vi "Control Drive Motors.vi"(10 "Disable Motors":bool=TRUE, 11 "Cluster":cluster{"RR":dbl, "FR":dbl, "RL":dbl, "FL":dbl}) -> ()   [LabVIEW 2018]
uses:
  <vilib>/Rock Robotics/WPI/Utilities/WPI_GetSetVariantRefNum.vi
  <vilib>/Rock Robotics/Network Tables/NT Write Number.vi
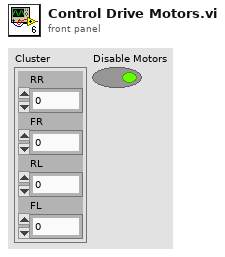
[diagram p1: front panel]
types:
  T1 = typedef "WPI_RobotDriveDevRef.ctl" = cluster{"DevStatus":errorcluster, "Motors[]":T2[], "Square Inputs":bool, "Max Output":dbl}
  T2 = typedef "WPI_MotorControlDeviceRef.ctl" = cluster{"DeviceStatus":errorcluster, "Type":T3, "PWM":cluster{"PWM Channel":T4, "DeadBand":T5}, "CAN":cluster{"Device Number":u8, "SetOutput VI Ref":variant, "GetOutput VI Ref":variant, "Enable VI Ref":variant, "Disable VI Ref":variant, "Data":variant}, "Invert":bool, "DIO PWM":cluster{"PWM \"Enable\" Channel":T4, "DIOChannel":T6, "PWM Rate":dbl}}
  T3 = typedef "WPI_MotorControlType.ctl" = enum16{"PWM", "CAN", "DIO PWM"}
  T4 = typedef "FPGA_DIOPWMChannel.ctl" = enum8{"PWM 0", "PWM 1", "PWM 2", "PWM 3", "PWM 4", "PWM 5", "PWM 6", "PWM 7", "PWM 8", "PWM 9", "PWM MXP 0", "PWM MXP 1", "PWM MXP 2", "PWM MXP 3", "PWM MXP 4", "PWM MXP 5", "PWM MXP 6", "PWM MXP 7", "PWM MXP 8", "PWM MXP 9", "Invalid"}
  T5 = typedef "WPI_PWMDeadband.ctl" = cluster{"Name":string, "maxPositivePwm":i32, "minPositivePwm":i32, "centerPwm":i32, "maxNegativePwm":i32, "minNegativePwm":i32, "angularRange":u16}
  T6 = typedef "FPGA_DIOChannel.ctl" = enum8{"DIO 0", "DIO 1", "DIO 2", "DIO 3", "DIO 4", "DIO 5", "DIO 6", "DIO 7", "DIO 8", "DIO 9", "DIO MXP 0", "DIO MXP 1", "DIO MXP 2", "DIO MXP 3", "DIO MXP 4", "DIO MXP 5", "DIO MXP 6", "DIO MXP 7", "DIO MXP 8", "DIO MXP 9", "DIO MXP 10", "DIO MXP 11", "DIO MXP 12", "DIO MXP 13", "DIO MXP 14", "DIO MXP 15", "SPI Port CS1", "SPI Port CS2", "SPI Port CS3", "SPI Port MISO", "SPI Port MOSI", "Invalid"}
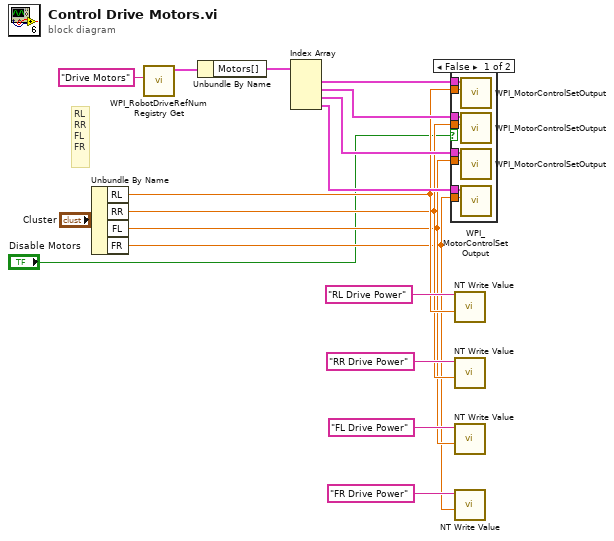
[diagram p0: block diagram]
diagram:
  # "RL\nRR\nFL\nFR"
  n1 = Unbundle By Name("Cluster") -> ("RL"=w5:dbl, "RR"=w4:dbl, "FL"=w3:dbl, "FR"=w2:dbl)
  n2 = call <vilib>:"WPI_RobotDriveRefNum Registry Get.vi"("refnum name"="Drive Motors") -> ("RobotDriveDevRef"=w17:T1)  [unwired: 9 in, 1 out]
  n3 = Unbundle By Name(w17) -> ("Motors[]"=w15:T2[])
  n4 = Index Array(array=w15) -> (element #1=w14:T2, element #2=w13:T2, element #3=w12:T2, element #4=w11:T2)  [unwired: 4 in]
  n5 = case shown="False" "Disable Motors" {
    tunnel: w14 -> [w25 _]
    tunnel: w13 -> [w24 _]
    tunnel: w12 -> [w23 _]
    tunnel: w11 -> [w22 _]
    tunnel: w5 -> [w21 _]
    tunnel: w4 -> [w20 _]
    tunnel: w3 -> [w19 _]
    tunnel: w2 -> [w18 _]
    frame False {
      n6 = call <vilib>:"WPI_MotorControlSetOutput.vi"("Output"=w21, "MotorControlDevRef"=w25) -> ()  [unwired: 7 in, 3 out]
      n7 = call <vilib>:"WPI_MotorControlSetOutput.vi"("Output"=w20, "MotorControlDevRef"=w24) -> ()  [unwired: 7 in, 3 out]
      n8 = call <vilib>:"WPI_MotorControlSetOutput.vi"("Output"=w19, "MotorControlDevRef"=w23) -> ()  [unwired: 7 in, 3 out]
      n9 = call <vilib>:"WPI_MotorControlSetOutput.vi"("Output"=w18, "MotorControlDevRef"=w22) -> ()  [unwired: 7 in, 3 out]
    }
    frame True {
    }
  }
  n10 = call-poly <vilib>:"NT Write Value.vi"("Numeric"=w5, "Name"="RL Drive Power") -> ()  [unwired: 9 in, 1 out]
  n11 = call-poly <vilib>:"NT Write Value.vi"("Numeric"=w4, "Name"="RR Drive Power") -> ()  [unwired: 9 in, 1 out]
  n12 = call-poly <vilib>:"NT Write Value.vi"("Numeric"=w3, "Name"="FL Drive Power") -> ()  [unwired: 9 in, 1 out]
  n13 = call-poly <vilib>:"NT Write Value.vi"("Numeric"=w2, "Name"="FR Drive Power") -> ()  [unwired: 9 in, 1 out]
